vi "RealSense_HelloWorld_PointCloud_ext_RGB2.vi"() -> ()   [LabVIEW 2019]
doc: "Simple Demo showing how to connect a RealSense Camera to stream COLOR and DEPTH from the stereo camera of a D4xx series camera."
uses:
  <vilib>/Utility/miscctls.llb/LV3DPointTypeDef.ctl
  <vilib>/Utility/miscctls.llb/LVRGBAColorTypeDef.ctl
  <vilib>/picture/3D Picture Control/Object/Create Object (name).vi
  Program Files (x86)/RealSense for Labview/RealSense for Labview ver. 2.33/libRealSense3.lvlib
  <vilib>/picture/3D Picture Control/NI_3D Picture Control.lvlib
panel:
  in  "Display tab":T1(tab)=enum."Color + Depth"
  out "RGB height":i32=720
  out "RGB width":i32=1280
  in  "Select RGB Resolution":u16(ring)=28 items=["424 x 240 @6fps", "424 x 240 @15fps", "424 x 240 @30fps", "424 x 240 @60fps", "640 x 480 @6fps", "640 x 480 @15fps", "640 x 480 @30fps", "1280 x 720 @6fps", "1280 x 720 @10fps", "1280 x 720 @15fps", "1920 x 1080 @8fps"]
  out "Depth height":i32=720
  out "Depth width":i32=1280
  out "init results":T2={"camera name"="Intel RealSense D435I", "camera S/N"="834412070342", "F/W"="05.12.01.00", "Sensor name"="Stereo Module", "api_version"=23201, "rscontext"=1659248689968, "device_list"=1659375430384, "device count"=1, "Dev out"=1659375543056, "sensor_list"=1659375327152, "sensor count"=3, "Sensor out"=1659374593968}
  in  "Select Depth Resolution":u16(ring)=29 items=["256 x 144 @90fps", "480 x 270 @6fps", "480 x 270 @15fps", "480 x 270 @30fps", "480 x 270 @60fps", "640 x 360 @30fps", "640 x 480 @6fps", "640 x 480 @15fps", "640 x 480 @30fps", "848 x 480 @6fps", "848 x 480 @8fps", "848 x 480 @10fps", "1280 x 720 @6fps"]
  in  "Sensor index":i32
  in  "Device index":i32
  out "L-R Baseline, mm":sgl=-49.906834
  out "fy":sgl=656.61536 format="%#_5g"
  out "fx":sgl=656.61536 format="%#_5g"
  out "ppy":sgl=357.01468 format="%#_5g"
  out "ppx":sgl=632.28015 format="%#_5g"
  out "RGB Sensor":T3={"Sensor info"="RGB Camera", "Sensor out"=1659374594288, "error"=0}
  out "Stream Profile Handles":u64[](array[numeric])=[1659375449352]
  out "queue out":u64=1659245873280
  out "sensor out":u64=1659374594288
  out "Sensor out":u64=1659374594288
  out "Stream type":u16(ring)=2 items=["Depth"=0, "Color (ext.)"=2, "Color (left) "=3, "IR Left"=5, "IR Right"=9, "IR Left (Y16)"=21, "IR Right (Y16)"=25]
  in  "Exposure,us":sgl=33000.0
  in  "Autoexposure":bool=TRUE
  in  "Depth Presets":T4(ring)=enum."Short Range"
  in  "Color Presets":T5(ring)=enum."D435"
  in  "Laser on/off":bool=TRUE
  in  "Gain(16-248)":sgl=30.0 min=16 max=248
  in  "Update Presets":bool
  in  "Laser \nPower (mW)":dbl(slide)=155.72448 min=0.0 max=360.0 scale=0.36..360.0
  in  "Range Scale":enum16{"200m", "100m", "60m", "6m", "2m", "1m"}(ring)=enum."6m"
  out "RGB image":picture
  out "Depth map":sgl[][](graph)
  out "3D Picture":refnum<vi>(3d-picture)
  out "init error":string="\rNo Error\rNo Error\rNo Error\rNo Error\rNo Error\rNo Error\rNo Error\r\rNo Error\rNo Error"
  out "iteration":i32=762
  in  "stop":bool=TRUE
  # "RealSense Hello World: PointCloud ext. RGB"
  # "This demo shows how to connect a RealSense D435 & D415 Stereo Depth Camera, and display the textured PointCloud."
  # "Note; When you change Depth Preset you need to stop and restart for the HDAD settings to take effect.\n\nTry the Color preset called \"Remove IR2\". It will remove the laser projector from the RGB 1280x720 image."
  # "INTRINSICS & EXTRINSICS"
  # "SELECT THE RESOLUTION"
  # "DEPTH MAP"
  # "COLOR"
  # "Changes Color scale for Depth Map."
  # "20-1660000"
  # "3D POINTCLOUD"
  # "Rotate: Drag image\nMove X-Y: HOLD DOWN CTRL while dragging.\nZoom: SHIFT while dragging."
  # "ERRORS"
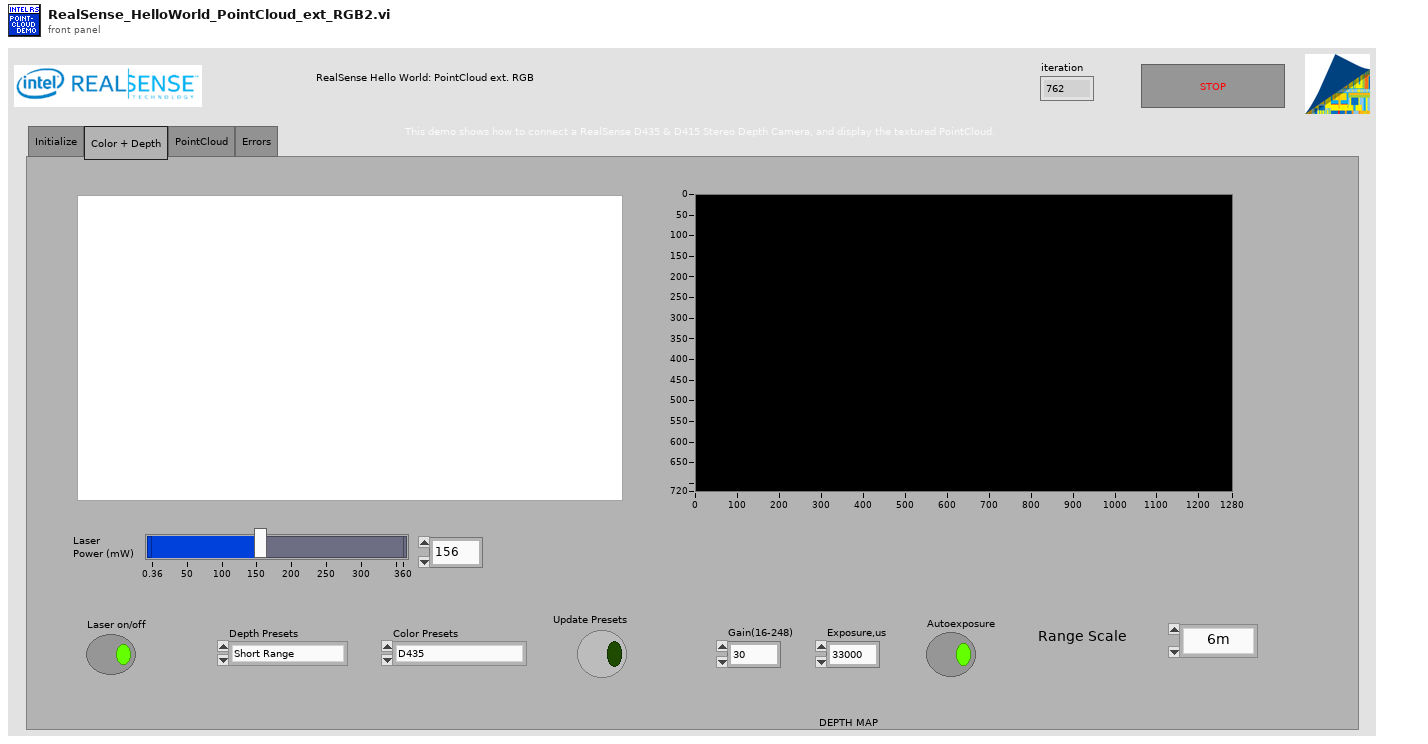
[diagram p1: front panel]
types:
  T1 = enum32{"Initialize", "Color + Depth", "PointCloud", "Errors"}
  T2 = cluster{"camera name":string, "camera S/N":string, "F/W":string, "Sensor name":string, "api_version":i32, "rscontext":u64, "device_list":u64, "device count":i32, "Dev out":u64, "sensor_list":u64, "sensor count":i32, "Sensor out":u64}
  T3 = cluster{"Sensor info":string, "Sensor out":u64, "error":u64}
  T4 = enum16{"Custom", "Original", "New Depth 1", "New Depth 2", "Depth Active 1", "Active 3D Scan", "Active Short A", "Active Short C", "Face", "Face2", "Best Box", "High Density", "Medium Density", "High Accuracy", "Hand", "Short Range", "Flat wall", "Load .JSON", "Load .JSON2"}
  T5 = enum16{"Custom", "RS400 (DS5p)", "RS400 (DS5p) 2", "RS400 (DS5p) 3", "RS400 (DS5p) 4", "RS400 (DS5p) 5", "RS410 (DS5a)", "RS410 (DS5a) 2", "DS410 (DS5a) 3", "DS410 (DS5a) 4", "DS410+IR", "DS5LR", "DS5LR-2", "DS5LR no pattern", "RS410 Remove IR", "RS410 Remove IR 2", "DS5micro", "D435"}
  T6 = cluster{"Sensor info":string, "Sensor out":u64, "error":u64}[]
  T7 = cluster{"width":i32, "height":i32, "fps":i32, "Profile":u64, "ppx":sgl, "ppy":sgl, "fx":sgl, "fy":sgl, "model":u32}
  T8 = enum16{"Overall", "Per Primitive", "Per Vertex", "Binding Off"}
  T9 = enum16{"Points", "Lines", "Line Strip", "Line Loop", "Triangles", "Triangle Strip", "Triangle Fan", "Quads", "Quad Strip", "Polygon"}
  T10 = cluster{"R":dbl, "G":dbl, "B":dbl, "Alpha":dbl}[]
  T11 = typedef "LVRGBAColorTypeDef.ctl" = cluster{"Red":sgl, "Green":sgl, "Blue":sgl, "Alpha":sgl}
  T12 = typedef "LV3DPointTypeDef.ctl" = cluster{"X":sgl, "Y":sgl, "Z":sgl}
  T13 = cluster{"Alpha":sgl, "Blue":sgl, "Green":sgl, "Red":sgl}
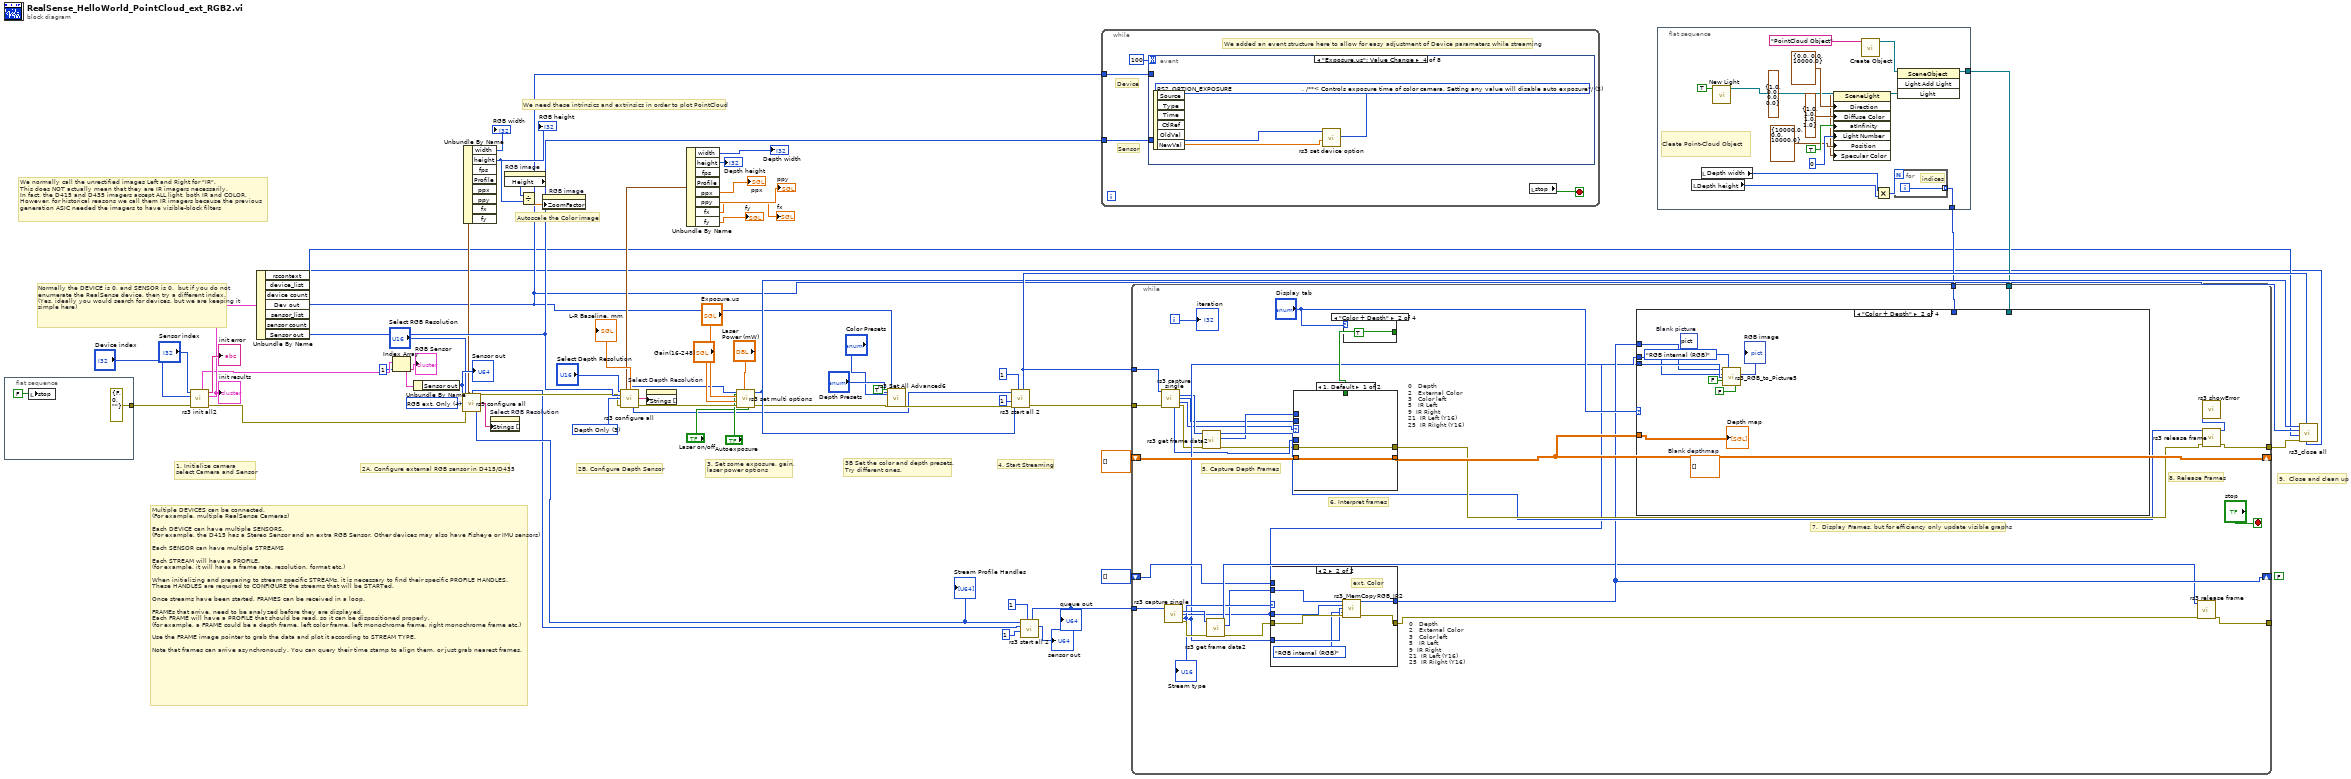
[diagram p0: block diagram]
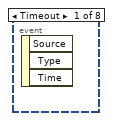
[diagram p2: hidden frame]
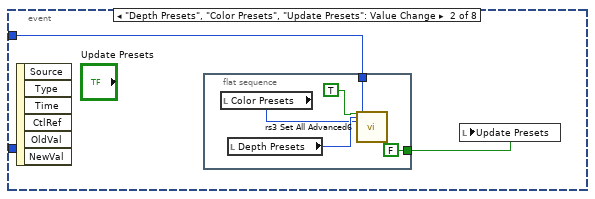
[diagram p3: hidden frame]
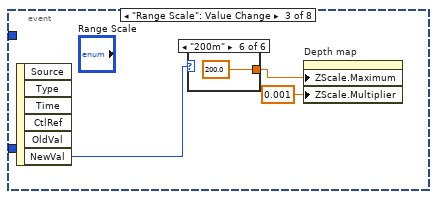
[diagram p4: hidden frame]
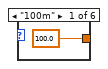
[diagram p5: hidden frame]
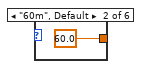
[diagram p6: hidden frame]
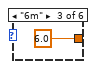
[diagram p7: hidden frame]
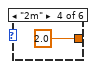
[diagram p8: hidden frame]
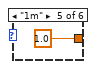
[diagram p9: hidden frame]
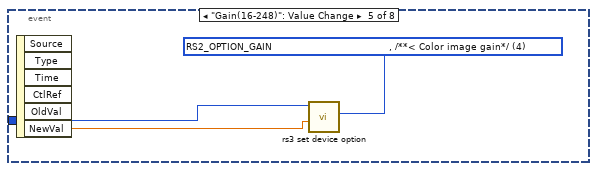
[diagram p10: hidden frame]
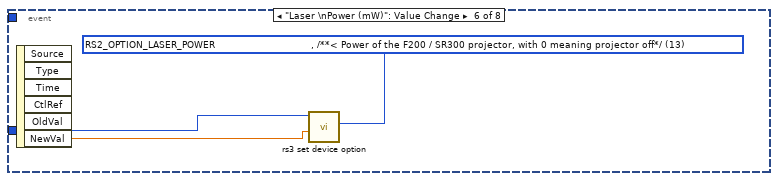
[diagram p11: hidden frame]
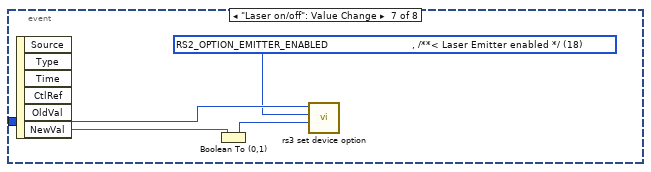
[diagram p12: hidden frame]
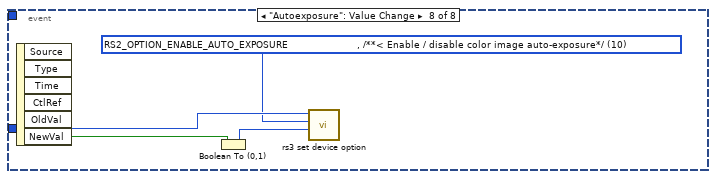
[diagram p13: hidden frame]
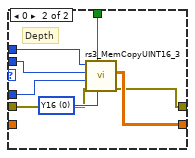
[diagram p14: hidden frame]
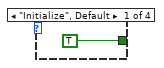
[diagram p16: hidden frame]
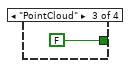
[diagram p17: hidden frame]
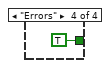
[diagram p18: hidden frame]
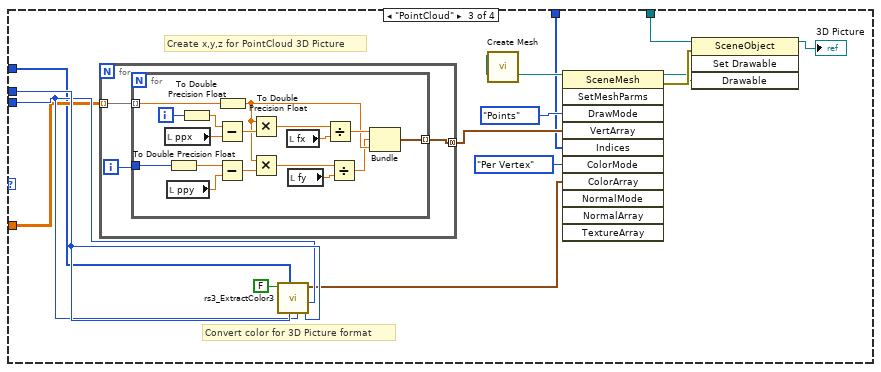
[diagram p20: hidden frame]
diagram:
  (unwired) FALSE
  w16 = u16 4 items=["Depth + Left Color", "Unrectified L + R", "Rectified L + R", "Depth Only", "RGB ext. Only"] ("Stream selection")
  w53 = u16 3 items=["Depth + Left Color", "Unrectified L + R", "Rectified L + R", "Depth Only", "RGB ext. Only"] ("Stream selection")
  # "2A. Configure external RGB sensor in D415/D435"
  # "Autoscale the Color image"
  # "We need these intrinsics and extrinsics in order to plot PointCloud"
  # "3B Set the color and depth presets.\nTry different ones."
  # "We normally call the unrectified images Left and Right for \"IR\". \nThis does NOT actually mean that they are IR imagers necessarily. \nIn fact, the D415 and D435 imagers accept ALL light, both IR and COLOR.\nHowever, for historical reasons we call them IR imagers because the previous generation ASIC needed the imagers to have visible-block filters"
  # "Normally the DEVICE is 0, and SENSOR is 0,  but if you do not enumerate the RealSense device, then try a different index.\n(Yes, ideally you would search for devices, but we are keeping it simple here)"
  # "Multiple DEVICES can be connected. \n(For example, multiple RealSense Cameras)\n\nEach DEVICE can have multiple SENSORS. \n(For example, the D415 has a Stereo Sensor and an extra RGB Sensor. Other devices may also have Fisheye or IMU sensors) \n\nEach SENSOR can have multiple STREAMS\n\nEach STREAM will have a PROFILE. \n(for example, it will have a frame rate, resolution, format etc.)\n\nWhen initializing and preparing to stream specific STREAMs, it is necessary to find their specific PROFILE HANDLES.\nThese HANDLES are required to CONFIGURE the streams that will be STARTed. \n\nOnce streams have been started, FRAMES can be received in a loop. \n \nFRAMEs that arrive, need to be analyzed before they are displayed. \nEach FRAME will have a PROFILE that should be read, so it can be dispositioned properly.\n(for example, a FRAME could be a depth frame, left color frame, left monochrome frame, right monochrome frame etc.)\n\nUse the FRAME image pointer to grab the data and plot it according to STREAM TYPE.\n\nNote that frames can arrive asynchronously. You can query their time stamp to align them, or just grab nearest frames."
  # "9.  Close and clean up"
  # "4. Start Streaming"
  # "3. Set some exposure, gain, \nlaser power options"
  # "2B. Configure Depth Sensor"
  # "1. Initialize camera\nselect Camera and Sensor"
  n1 = flat-sequence {
    tunnel: [errorcluster {"status"=FALSE, "code"=0, "source"=""} ("error in")] -> w54
    frame #0 {
      n2 = local write "stop"(FALSE ("stop")) -> ()
    }
  }
  n3 = call "rs3 init all2.vi"("error in"=w54, "Select Device"="Device index", "Select Sensor"="Sensor index") -> ("error out"=w22:errorcluster, "init results"=w58:T2, "init error"=→"init error":string, "Sensor Array"=w26:T6)  [unwired: 2 in, 3 out]
  "init results" <- w58
  n4 = Unbundle By Name(w58) -> ("rscontext"=w4:u64, "device_list"=w6:u64, "Dev out"=w7:u64, "Sensor out"=w41:u64)  [unwired: 3 out]
  n5 = Index Array(array=w26, index=1) -> (element=w24:T3)
  "RGB Sensor" <- w24
  n6 = Unbundle By Name(w24) -> ("Sensor out"=w23:u64)
  "Sensor out" <- w23
  n7 = call "rs3 configure all.vi"("Select Resolution"="Select RGB Resolution", "Sensor in"=w23, "Stream selection"=w16, "error in (no error)"=w22) -> ("Output stream L"=w19:T7, "Sensor out"=w13:u64, "Output stream"=w3:string[], "Stream Profile Handles"=w14:u64[], "error out"=w20:errorcluster)  [unwired: 2 in, 5 out]
  "Stream Profile Handles" <- w14
  n8 = Unbundle By Name(w19) -> ("width"=→"RGB width":i32, "height"=w17:i32)  [unwired: 6 out]
  "RGB height" <- w17
  n9 = property on="Select RGB Resolution" class="Ring (strict)"("Strings []"=w3) -> ()  [unwired: 2 in, 2 out]
  n10 = property on="RGB image" class="Pict"() -> ("Height"=w37:u32)  [unwired: 2 in, 2 out]
  n11 = Divide(x=w37, y=w17) -> (x/y=w35:dbl)
  n12 = property on="RGB image" class="Pict"("ZoomFactor"=w35) -> ()  [unwired: 2 in, 2 out]
  n13 = call "rs3 configure all.vi"("Select Resolution"="Select Depth Resolution", "Sensor in"=w41, "Stream selection"=w53, "error in (no error)"=w20) -> ("Output stream L"=w38:T7, "Sensor out"=w27:u64, "Output stream"=w55:string[], "L-R Baseline, mm"=→"L-R Baseline, mm":sgl, "Stream Profile Handles"=w15:u64[], "error out"=w52:errorcluster)  [unwired: 2 in, 4 out]
  n14 = property on="Select Depth Resolution" class="Ring (strict)"("Strings []"=w55) -> ()  [unwired: 2 in, 2 out]
  n15 = Unbundle By Name(w38) -> ("width"=→"Depth width":i32, "height"=→"Depth height":i32, "ppx"=→"ppx":sgl, "ppy"=→"ppy":sgl, "fx"=→"fx":sgl, "fy"=→"fy":sgl)  [unwired: 2 out]
  n16 = call "rs3 set multi options.vi"("laser on/off"="Laser on/off", "autoexposure"="Autoexposure", "Laser power, mW (0-360)"="Laser \nPower (mW)", "error in (no error)"=w52, "Gain(16-248)"="Gain(16-248)", "Exposure, us"="Exposure,us", "Sensor in"=w27) -> ("error out"=w46:errorcluster, "Sensor out"=w51:u64)  [unwired: 2 in, 1 out]
  n17 = call "rs3 Set All Advanced6.vi"("Set Color Corr"=TRUE, "Depth Presets"="Depth Presets", "Color Presets"="Color Presets", "error in (no error)"=w46, "device in"=w7) -> ("error out"=w45:errorcluster)  [unwired: 20 in, 2 out]
  n18 = call "rs3 start all 2.vi"("capacity"=1, "error in (no error)"=w45, "Count of Streams"=1, "Sensor in"=w51, "Stream profile array"=w15) -> ("error out"=w56:errorcluster, "queue out"=w61:u64)  [unwired: 3 in, 2 out]
  n19 = call "rs3 start all 2.vi"("capacity"=1, "Count of Streams"=1, "Sensor in"=w13, "Stream profile array"=w14) -> ("sensor out"=→"sensor out":u64, "queue out"=w5:u64)  [unwired: 4 in, 2 out]
  "queue out" <- w5
  n20 = while {
    tunnel: w7 -> [w68]
    tunnel: w41 -> [w67]
    stop <- w69 stop-if-true
    # "Sensor"
    # "Device"
    # "We added an event structure here to allow for easy adjustment of Device parameters while streaming"
    n21 = event shown="[3] \"Exposure,us\": Value Change" {
      selector: _ -> [_ _ _ _ _ _ _ _]
      dyn-events: _ -> [_ _ _ _ _ _ _ _]
      timeout: 100 -> [_ _ _ _ _ _ _ _]
      tunnel: w68 -> [_ w71 _ _ _ _ _ _]
      tunnel: w67 -> [_ _ _ w88 w91 w94 w98 w102]
      event Timeout {
        n22 = event-data() -> ()  [unwired: 1 in, 3 out]
      }
      event "Depth Presets", "Color Presets", "Update Presets": Value Change {
        n23 = event-data() -> ()  [unwired: 1 in, 6 out]
        n24 = flat-sequence {
          tunnel: w71 -> [w73]
          tunnel: [FALSE ("Update Presets")] -> w70
          frame #0 {
            n25 = local read "Color Presets"() -> (w75:T5)
            n26 = local read "Depth Presets"() -> (w76:T4)
            n27 = call "rs3 Set All Advanced6.vi"("Set Color Corr"=TRUE, "Depth Presets"=w76, "Color Presets"=w75, "device in"=w73) -> ()  [unwired: 21 in, 3 out]
          }
        }
        n28 = local write "Update Presets"(w70) -> ()
      }
      event "Range Scale": Value Change {
        n29 = event-data() -> ("NewVal"=w78:enum16{"200m", "100m", "60m", "6m", "2m", "1m"})  [unwired: 1 in, 5 out]
        n30 = case shown="\"200m\"" w78 {
          tunnel: [100.0 ("Z Scale.Offset and Multiplier:Multiplier") 60.0 ("Z Scale.Offset and Multiplier:Multiplier") 6.0 ("Z Scale.Offset and Multiplier:Multiplier") 2.0 ("Z Scale.Offset and Multiplier:Multiplier") 1.0 ("Z Scale.Offset and Multiplier:Multiplier") 200.0 ("Z Scale.Offset and Multiplier:Multiplier")] -> w77
          frame "100m" {
          }
          frame "60m", Default {
          }
          frame "6m" {
          }
          frame "2m" {
          }
          frame "1m" {
          }
          frame "200m" {
          }
        }
        n31 = property on="Depth map" class="IntGraph (strict)"("ZScale.Maximum"=w77, "ZScale.Multiplier"=0.001 ("Z Scale.Offset and Multiplier:Multiplier")) -> ()  [unwired: 2 in, 2 out]
      }
      event "Exposure,us": Value Change {
        w86 = u16 3 items=["    RS2_OPTION_BACKLIGHT_COMPENSATION                     , /**< Enable / disable color backlight compensation*/", "    RS2_OPTION_BRIGHTNESS                                 , /**< Color image brightness*/", "    RS2_OPTION_CONTRAST                                   , /**< Color image contrast*/", "    RS2_OPTION_EXPOSURE                                   , /**< Controls exposure time of color camera. Setting any value will disable auto exposure*/", "    RS2_OPTION_GAIN                                       , /**< Color image gain*/", "    RS2_OPTION_GAMMA                                      , /**< Color image gamma setting*/", "    RS2_OPTION_HUE                                        , /**< Color image hue*/", "    RS2_OPTION_SATURATION                                 , /**< Color image saturation setting*/", "    RS2_OPTION_SHARPNESS                                  , /**< Color image sharpness setting*/", "    RS2_OPTION_WHITE_BALANCE                              , /**< Controls white balance of color image. Setting any value will disable auto white balance*/", "    RS2_OPTION_ENABLE_AUTO_EXPOSURE                       , /**< Enable / disable color image auto-exposure*/", "    RS2_OPTION_ENABLE_AUTO_WHITE_BALANCE                  , /**< Enable / disable color image auto-white-balance*/", "    RS2_OPTION_VISUAL_PRESET                              , /**< Provide access to several recommend sets of option presets for the depth camera */", "    RS2_OPTION_LASER_POWER                                , /**< Power of the F200 / SR300 projector, with 0 meaning projector off*/", "    RS2_OPTION_ACCURACY                                   , /**< Set the number of patterns projected per frame. The higher the accuracy value the more patterns projected. Increasing the number of patterns help to achieve better accuracy. Note that this c", "    RS2_OPTION_MOTION_RANGE                               , /**< Motion vs. Range trade-off, with lower values allowing for better motion sensitivity and higher values allowing for better depth range*/", "    RS2_OPTION_FILTER_OPTION                              , /**< Set the filter to apply to each depth frame. Each one of the filter is optimized per the application requirements*/", "    RS2_OPTION_CONFIDENCE_THRESHOLD                       , /**< The confidence level threshold used by the Depth algorithm pipe to set whether a pixel will get a valid range or will be marked with invalid range*/", "    RS2_OPTION_EMITTER_ENABLED                            , /**< Laser Emitter enabled */", "    RS2_OPTION_FRAMES_QUEUE_SIZE                          , /**< Number of frames the user is allowed to keep per stream. Trying to hold-on to more frames will cause frame-drops.*/", "    RS2_OPTION_TOTAL_FRAME_DROPS                          , /**< Total number of detected frame drops from all streams */", "    RS2_OPTION_AUTO_EXPOSURE_MODE                         , /**< Auto-Exposure modes: Static, Anti-Flicker and Hybrid */", "    RS2_OPTION_POWER_LINE_FREQUENCY                       , /**< Power Line Frequency control for anti-flickering Off/50Hz/60Hz/Auto */", "    RS2_OPTION_ASIC_TEMPERATURE                           , /**< Current Asic Temperature */", "    RS2_OPTION_ERROR_POLLING_ENABLED                      , /**< disable error handling */", "    RS2_OPTION_PROJECTOR_TEMPERATURE                      , /**< Current Projector Temperature */", "    RS2_OPTION_OUTPUT_TRIGGER_ENABLED                     , /**< Enable / disable trigger to be outputed from the camera to any external device on every depth frame */", "    RS2_OPTION_MOTION_MODULE_TEMPERATURE                  , /**< Current Motion-Module Temperature */", "    RS2_OPTION_DEPTH_UNITS                                , /**< Number of meters represented by a single depth unit */", "    RS2_OPTION_ENABLE_MOTION_CORRECTION                   , /**< Enable/Disable automatic correction of the motion data */", "    RS2_OPTION_AUTO_EXPOSURE_PRIORITY                     , /**< Allows sensor to dynamically ajust the frame rate depending on lighting conditions */", "    RS2_OPTION_COUNT                                      , /**< Number of enumeration values. Not a valid input: intended to be used in for-loops. */"] ("RS Option")
        n32 = event-data() -> ("NewVal"=w87:sgl)  [unwired: 1 in, 5 out]
        n33 = call "rs3 set device option.vi"("value"=w87, "RS Option"=w86, "Sensor in"=w88) -> ()  [unwired: 6 in, 3 out]
      }
      event "Gain(16-248)": Value Change {
        w89 = u16 4 items=["    RS2_OPTION_BACKLIGHT_COMPENSATION                     , /**< Enable / disable color backlight compensation*/", "    RS2_OPTION_BRIGHTNESS                                 , /**< Color image brightness*/", "    RS2_OPTION_CONTRAST                                   , /**< Color image contrast*/", "    RS2_OPTION_EXPOSURE                                   , /**< Controls exposure time of color camera. Setting any value will disable auto exposure*/", "    RS2_OPTION_GAIN                                       , /**< Color image gain*/", "    RS2_OPTION_GAMMA                                      , /**< Color image gamma setting*/", "    RS2_OPTION_HUE                                        , /**< Color image hue*/", "    RS2_OPTION_SATURATION                                 , /**< Color image saturation setting*/", "    RS2_OPTION_SHARPNESS                                  , /**< Color image sharpness setting*/", "    RS2_OPTION_WHITE_BALANCE                              , /**< Controls white balance of color image. Setting any value will disable auto white balance*/", "    RS2_OPTION_ENABLE_AUTO_EXPOSURE                       , /**< Enable / disable color image auto-exposure*/", "    RS2_OPTION_ENABLE_AUTO_WHITE_BALANCE                  , /**< Enable / disable color image auto-white-balance*/", "    RS2_OPTION_VISUAL_PRESET                              , /**< Provide access to several recommend sets of option presets for the depth camera */", "    RS2_OPTION_LASER_POWER                                , /**< Power of the F200 / SR300 projector, with 0 meaning projector off*/", "    RS2_OPTION_ACCURACY                                   , /**< Set the number of patterns projected per frame. The higher the accuracy value the more patterns projected. Increasing the number of patterns help to achieve better accuracy. Note that this c", "    RS2_OPTION_MOTION_RANGE                               , /**< Motion vs. Range trade-off, with lower values allowing for better motion sensitivity and higher values allowing for better depth range*/", "    RS2_OPTION_FILTER_OPTION                              , /**< Set the filter to apply to each depth frame. Each one of the filter is optimized per the application requirements*/", "    RS2_OPTION_CONFIDENCE_THRESHOLD                       , /**< The confidence level threshold used by the Depth algorithm pipe to set whether a pixel will get a valid range or will be marked with invalid range*/", "    RS2_OPTION_EMITTER_ENABLED                            , /**< Laser Emitter enabled */", "    RS2_OPTION_FRAMES_QUEUE_SIZE                          , /**< Number of frames the user is allowed to keep per stream. Trying to hold-on to more frames will cause frame-drops.*/", "    RS2_OPTION_TOTAL_FRAME_DROPS                          , /**< Total number of detected frame drops from all streams */", "    RS2_OPTION_AUTO_EXPOSURE_MODE                         , /**< Auto-Exposure modes: Static, Anti-Flicker and Hybrid */", "    RS2_OPTION_POWER_LINE_FREQUENCY                       , /**< Power Line Frequency control for anti-flickering Off/50Hz/60Hz/Auto */", "    RS2_OPTION_ASIC_TEMPERATURE                           , /**< Current Asic Temperature */", "    RS2_OPTION_ERROR_POLLING_ENABLED                      , /**< disable error handling */", "    RS2_OPTION_PROJECTOR_TEMPERATURE                      , /**< Current Projector Temperature */", "    RS2_OPTION_OUTPUT_TRIGGER_ENABLED                     , /**< Enable / disable trigger to be outputed from the camera to any external device on every depth frame */", "    RS2_OPTION_MOTION_MODULE_TEMPERATURE                  , /**< Current Motion-Module Temperature */", "    RS2_OPTION_DEPTH_UNITS                                , /**< Number of meters represented by a single depth unit */", "    RS2_OPTION_ENABLE_MOTION_CORRECTION                   , /**< Enable/Disable automatic correction of the motion data */", "    RS2_OPTION_AUTO_EXPOSURE_PRIORITY                     , /**< Allows sensor to dynamically ajust the frame rate depending on lighting conditions */", "    RS2_OPTION_COUNT                                      , /**< Number of enumeration values. Not a valid input: intended to be used in for-loops. */"] ("RS Option")
        n34 = event-data() -> ("NewVal"=w90:sgl)  [unwired: 1 in, 5 out]
        n35 = call "rs3 set device option.vi"("value"=w90, "RS Option"=w89, "Sensor in"=w91) -> ()  [unwired: 6 in, 3 out]
      }
      event "Laser \nPower (mW)": Value Change {
        w92 = u16 13 items=["    RS2_OPTION_BACKLIGHT_COMPENSATION                     , /**< Enable / disable color backlight compensation*/", "    RS2_OPTION_BRIGHTNESS                                 , /**< Color image brightness*/", "    RS2_OPTION_CONTRAST                                   , /**< Color image contrast*/", "    RS2_OPTION_EXPOSURE                                   , /**< Controls exposure time of color camera. Setting any value will disable auto exposure*/", "    RS2_OPTION_GAIN                                       , /**< Color image gain*/", "    RS2_OPTION_GAMMA                                      , /**< Color image gamma setting*/", "    RS2_OPTION_HUE                                        , /**< Color image hue*/", "    RS2_OPTION_SATURATION                                 , /**< Color image saturation setting*/", "    RS2_OPTION_SHARPNESS                                  , /**< Color image sharpness setting*/", "    RS2_OPTION_WHITE_BALANCE                              , /**< Controls white balance of color image. Setting any value will disable auto white balance*/", "    RS2_OPTION_ENABLE_AUTO_EXPOSURE                       , /**< Enable / disable color image auto-exposure*/", "    RS2_OPTION_ENABLE_AUTO_WHITE_BALANCE                  , /**< Enable / disable color image auto-white-balance*/", "    RS2_OPTION_VISUAL_PRESET                              , /**< Provide access to several recommend sets of option presets for the depth camera */", "    RS2_OPTION_LASER_POWER                                , /**< Power of the F200 / SR300 projector, with 0 meaning projector off*/", "    RS2_OPTION_ACCURACY                                   , /**< Set the number of patterns projected per frame. The higher the accuracy value the more patterns projected. Increasing the number of patterns help to achieve better accuracy. Note that this c", "    RS2_OPTION_MOTION_RANGE                               , /**< Motion vs. Range trade-off, with lower values allowing for better motion sensitivity and higher values allowing for better depth range*/", "    RS2_OPTION_FILTER_OPTION                              , /**< Set the filter to apply to each depth frame. Each one of the filter is optimized per the application requirements*/", "    RS2_OPTION_CONFIDENCE_THRESHOLD                       , /**< The confidence level threshold used by the Depth algorithm pipe to set whether a pixel will get a valid range or will be marked with invalid range*/", "    RS2_OPTION_EMITTER_ENABLED                            , /**< Laser Emitter enabled */", "    RS2_OPTION_FRAMES_QUEUE_SIZE                          , /**< Number of frames the user is allowed to keep per stream. Trying to hold-on to more frames will cause frame-drops.*/", "    RS2_OPTION_TOTAL_FRAME_DROPS                          , /**< Total number of detected frame drops from all streams */", "    RS2_OPTION_AUTO_EXPOSURE_MODE                         , /**< Auto-Exposure modes: Static, Anti-Flicker and Hybrid */", "    RS2_OPTION_POWER_LINE_FREQUENCY                       , /**< Power Line Frequency control for anti-flickering Off/50Hz/60Hz/Auto */", "    RS2_OPTION_ASIC_TEMPERATURE                           , /**< Current Asic Temperature */", "    RS2_OPTION_ERROR_POLLING_ENABLED                      , /**< disable error handling */", "    RS2_OPTION_PROJECTOR_TEMPERATURE                      , /**< Current Projector Temperature */", "    RS2_OPTION_OUTPUT_TRIGGER_ENABLED                     , /**< Enable / disable trigger to be outputed from the camera to any external device on every depth frame */", "    RS2_OPTION_MOTION_MODULE_TEMPERATURE                  , /**< Current Motion-Module Temperature */", "    RS2_OPTION_DEPTH_UNITS                                , /**< Number of meters represented by a single depth unit */", "    RS2_OPTION_ENABLE_MOTION_CORRECTION                   , /**< Enable/Disable automatic correction of the motion data */", "    RS2_OPTION_AUTO_EXPOSURE_PRIORITY                     , /**< Allows sensor to dynamically ajust the frame rate depending on lighting conditions */", "    RS2_OPTION_COUNT                                      , /**< Number of enumeration values. Not a valid input: intended to be used in for-loops. */"] ("RS Option")
        n36 = event-data() -> ("NewVal"=w93:dbl)  [unwired: 1 in, 5 out]
        n37 = call "rs3 set device option.vi"("value"=w93, "RS Option"=w92, "Sensor in"=w94) -> ()  [unwired: 6 in, 3 out]
      }
      event "Laser on/off": Value Change {
        w97 = u16 18 items=["    RS2_OPTION_BACKLIGHT_COMPENSATION                     , /**< Enable / disable color backlight compensation*/", "    RS2_OPTION_BRIGHTNESS                                 , /**< Color image brightness*/", "    RS2_OPTION_CONTRAST                                   , /**< Color image contrast*/", "    RS2_OPTION_EXPOSURE                                   , /**< Controls exposure time of color camera. Setting any value will disable auto exposure*/", "    RS2_OPTION_GAIN                                       , /**< Color image gain*/", "    RS2_OPTION_GAMMA                                      , /**< Color image gamma setting*/", "    RS2_OPTION_HUE                                        , /**< Color image hue*/", "    RS2_OPTION_SATURATION                                 , /**< Color image saturation setting*/", "    RS2_OPTION_SHARPNESS                                  , /**< Color image sharpness setting*/", "    RS2_OPTION_WHITE_BALANCE                              , /**< Controls white balance of color image. Setting any value will disable auto white balance*/", "    RS2_OPTION_ENABLE_AUTO_EXPOSURE                       , /**< Enable / disable color image auto-exposure*/", "    RS2_OPTION_ENABLE_AUTO_WHITE_BALANCE                  , /**< Enable / disable color image auto-white-balance*/", "    RS2_OPTION_VISUAL_PRESET                              , /**< Provide access to several recommend sets of option presets for the depth camera */", "    RS2_OPTION_LASER_POWER                                , /**< Power of the F200 / SR300 projector, with 0 meaning projector off*/", "    RS2_OPTION_ACCURACY                                   , /**< Set the number of patterns projected per frame. The higher the accuracy value the more patterns projected. Increasing the number of patterns help to achieve better accuracy. Note that this c", "    RS2_OPTION_MOTION_RANGE                               , /**< Motion vs. Range trade-off, with lower values allowing for better motion sensitivity and higher values allowing for better depth range*/", "    RS2_OPTION_FILTER_OPTION                              , /**< Set the filter to apply to each depth frame. Each one of the filter is optimized per the application requirements*/", "    RS2_OPTION_CONFIDENCE_THRESHOLD                       , /**< The confidence level threshold used by the Depth algorithm pipe to set whether a pixel will get a valid range or will be marked with invalid range*/", "    RS2_OPTION_EMITTER_ENABLED                            , /**< Laser Emitter enabled */", "    RS2_OPTION_FRAMES_QUEUE_SIZE                          , /**< Number of frames the user is allowed to keep per stream. Trying to hold-on to more frames will cause frame-drops.*/", "    RS2_OPTION_TOTAL_FRAME_DROPS                          , /**< Total number of detected frame drops from all streams */", "    RS2_OPTION_AUTO_EXPOSURE_MODE                         , /**< Auto-Exposure modes: Static, Anti-Flicker and Hybrid */", "    RS2_OPTION_POWER_LINE_FREQUENCY                       , /**< Power Line Frequency control for anti-flickering Off/50Hz/60Hz/Auto */", "    RS2_OPTION_ASIC_TEMPERATURE                           , /**< Current Asic Temperature */", "    RS2_OPTION_ERROR_POLLING_ENABLED                      , /**< disable error handling */", "    RS2_OPTION_PROJECTOR_TEMPERATURE                      , /**< Current Projector Temperature */", "    RS2_OPTION_OUTPUT_TRIGGER_ENABLED                     , /**< Enable / disable trigger to be outputed from the camera to any external device on every depth frame */", "    RS2_OPTION_MOTION_MODULE_TEMPERATURE                  , /**< Current Motion-Module Temperature */", "    RS2_OPTION_DEPTH_UNITS                                , /**< Number of meters represented by a single depth unit */", "    RS2_OPTION_ENABLE_MOTION_CORRECTION                   , /**< Enable/Disable automatic correction of the motion data */", "    RS2_OPTION_AUTO_EXPOSURE_PRIORITY                     , /**< Allows sensor to dynamically ajust the frame rate depending on lighting conditions */", "    RS2_OPTION_COUNT                                      , /**< Number of enumeration values. Not a valid input: intended to be used in for-loops. */"] ("RS Option")
        n38 = event-data() -> ("NewVal"=w96:bool)  [unwired: 1 in, 5 out]
        n39 = Boolean To (0,1)(Boolean=w96) -> (0, 1=w95:i16)
        n40 = call "rs3 set device option.vi"("value"=w95, "RS Option"=w97, "Sensor in"=w98) -> ()  [unwired: 6 in, 3 out]
      }
      event "Autoexposure": Value Change {
        w101 = u16 10 items=["    RS2_OPTION_BACKLIGHT_COMPENSATION                     , /**< Enable / disable color backlight compensation*/", "    RS2_OPTION_BRIGHTNESS                                 , /**< Color image brightness*/", "    RS2_OPTION_CONTRAST                                   , /**< Color image contrast*/", "    RS2_OPTION_EXPOSURE                                   , /**< Controls exposure time of color camera. Setting any value will disable auto exposure*/", "    RS2_OPTION_GAIN                                       , /**< Color image gain*/", "    RS2_OPTION_GAMMA                                      , /**< Color image gamma setting*/", "    RS2_OPTION_HUE                                        , /**< Color image hue*/", "    RS2_OPTION_SATURATION                                 , /**< Color image saturation setting*/", "    RS2_OPTION_SHARPNESS                                  , /**< Color image sharpness setting*/", "    RS2_OPTION_WHITE_BALANCE                              , /**< Controls white balance of color image. Setting any value will disable auto white balance*/", "    RS2_OPTION_ENABLE_AUTO_EXPOSURE                       , /**< Enable / disable color image auto-exposure*/", "    RS2_OPTION_ENABLE_AUTO_WHITE_BALANCE                  , /**< Enable / disable color image auto-white-balance*/", "    RS2_OPTION_VISUAL_PRESET                              , /**< Provide access to several recommend sets of option presets for the depth camera */", "    RS2_OPTION_LASER_POWER                                , /**< Power of the F200 / SR300 projector, with 0 meaning projector off*/", "    RS2_OPTION_ACCURACY                                   , /**< Set the number of patterns projected per frame. The higher the accuracy value the more patterns projected. Increasing the number of patterns help to achieve better accuracy. Note that this c", "    RS2_OPTION_MOTION_RANGE                               , /**< Motion vs. Range trade-off, with lower values allowing for better motion sensitivity and higher values allowing for better depth range*/", "    RS2_OPTION_FILTER_OPTION                              , /**< Set the filter to apply to each depth frame. Each one of the filter is optimized per the application requirements*/", "    RS2_OPTION_CONFIDENCE_THRESHOLD                       , /**< The confidence level threshold used by the Depth algorithm pipe to set whether a pixel will get a valid range or will be marked with invalid range*/", "    RS2_OPTION_EMITTER_ENABLED                            , /**< Laser Emitter enabled */", "    RS2_OPTION_FRAMES_QUEUE_SIZE                          , /**< Number of frames the user is allowed to keep per stream. Trying to hold-on to more frames will cause frame-drops.*/", "    RS2_OPTION_TOTAL_FRAME_DROPS                          , /**< Total number of detected frame drops from all streams */", "    RS2_OPTION_AUTO_EXPOSURE_MODE                         , /**< Auto-Exposure modes: Static, Anti-Flicker and Hybrid */", "    RS2_OPTION_POWER_LINE_FREQUENCY                       , /**< Power Line Frequency control for anti-flickering Off/50Hz/60Hz/Auto */", "    RS2_OPTION_ASIC_TEMPERATURE                           , /**< Current Asic Temperature */", "    RS2_OPTION_ERROR_POLLING_ENABLED                      , /**< disable error handling */", "    RS2_OPTION_PROJECTOR_TEMPERATURE                      , /**< Current Projector Temperature */", "    RS2_OPTION_OUTPUT_TRIGGER_ENABLED                     , /**< Enable / disable trigger to be outputed from the camera to any external device on every depth frame */", "    RS2_OPTION_MOTION_MODULE_TEMPERATURE                  , /**< Current Motion-Module Temperature */", "    RS2_OPTION_DEPTH_UNITS                                , /**< Number of meters represented by a single depth unit */", "    RS2_OPTION_ENABLE_MOTION_CORRECTION                   , /**< Enable/Disable automatic correction of the motion data */", "    RS2_OPTION_AUTO_EXPOSURE_PRIORITY                     , /**< Allows sensor to dynamically ajust the frame rate depending on lighting conditions */", "    RS2_OPTION_COUNT                                      , /**< Number of enumeration values. Not a valid input: intended to be used in for-loops. */"] ("RS Option")
        n41 = event-data() -> ("NewVal"=w100:bool)  [unwired: 1 in, 5 out]
        n42 = Boolean To (0,1)(Boolean=w100) -> (0, 1=w99:i16)
        n43 = call "rs3 set device option.vi"("value"=w99, "RS Option"=w101, "Sensor in"=w102) -> ()  [unwired: 6 in, 3 out]
      }
    }
    n44 = local read "stop"() -> (w69:bool)
  }
  n45 = while {
    tunnel: w61 -> [w133]
    tunnel: w56 -> [w136]
    tunnel: [w134] -> w60
    shift-right: [w126] -> _
    shift-left: sgl[][] [] ("2D Array Output") -> [w131]
    tunnel: w30 -> [w130]
    tunnel: w28 -> [w129]
    tunnel: w5 -> [w123]
    tunnel: [w118] -> _
    shift-right: [w117] -> _
    shift-left: u8[] [] ("Output Array") -> [w115]
    i -> [w135]
    stop <- "stop" stop-if-true
    # "0   Depth\n2   External Color \n3   Color left\n5   IR Left \n9  IR Right\n21  IR Left (Y16)\n25  IR RiIght (Y16)"
    # "0   Depth\n2   External Color \n3   Color left\n5   IR Left \n9  IR Right\n21  IR Left (Y16)\n25  IR RiIght (Y16)"
    # "6. Interpret frames"
    # "5. Capture Depth Frames"
    # "8. Release Frames"
    # "7.  Display Frames, but for efficiency only update visible graphs"
    n46 = call "rs3 capture single.vi"("queue in"=w133, "error in (no error)"=w136) -> ("frame out"=w110:u64, "width"=w107:i32, "Stream type"=w108:u16, "height"=w106:i32, "error out"=w104:errorcluster)  [unwired: 5 in, 4 out]
    n47 = call "rs3 capture single.vi"("queue in"=w123) -> ("frame out"=w121:u64, "width"=w112:i32, "Stream type"=w114:u16, "height"=w111:i32, "error out"=w122:errorcluster)  [unwired: 6 in, 4 out]
    "Stream type" <- w114
    n48 = call "rs3 get frame data2.vi"("error in (no error)"=w104, "frame in"=w110) -> ("error out"=w105:errorcluster, "image pointer out"=w109:u64, "Frame out"=w124:u64)  [unwired: 6 in, 1 out]
    n49 = call "rs3 get frame data2.vi"("error in (no error)"=w122, "frame in"=w121) -> ("error out"=w120:errorcluster, "image pointer out"=w113:u64, "Frame out"=w116:u64)  [unwired: 6 in, 1 out]
    n50 = case shown="2" w114 {
      tunnel: [w148 w154] -> w119
      tunnel: w113 -> [_ w155]
      tunnel: w120 -> [w148 w153]
      tunnel: w112 -> [_ w152]
      tunnel: w111 -> [_ w151]
      tunnel: [w147 w150] -> w117
      tunnel: w115 -> [w147 _]
      frame 1, Default {
      }
      frame 2 {
        # "ext. Color"
        n51 = call "rs3_MemCopyRGB_IR2.vi"("Zimage pointer"=w155, "RGB  X, width"=w152, "RGB Y, height"=w151, "Color format"=enum16{"Monochrome", "RGB internal (RGB)"}."RGB internal (RGB)", "error in (no error)"=w153) -> ("Output Array"=w150:u8[], "error out"=w154:errorcluster)  [unwired: 8 in, 1 out]
      }
    }
    n52 = case shown="\"Color + Depth\"" "Display tab" {
      tunnel: [TRUE ("Transpose") TRUE ("Transpose") FALSE ("Transpose") TRUE ("Transpose")] -> w127
      frame "Initialize", Default {
      }
      frame "Color + Depth" {
      }
      frame "PointCloud" {
      }
      frame "Errors" {
      }
    }
    n53 = case shown="1, Default" w108 {
      tunnel: [w138 w143] -> w125
      tunnel: w109 -> [_ w142]
      tunnel: w107 -> [_ w141]
      tunnel: w106 -> [_ w140]
      tunnel: w105 -> [w138 w144]
      tunnel: [w137 w145] -> w126
      tunnel: w131 -> [w137 _]
      tunnel: w127 -> [_ w139]
      frame 1, Default {
      }
      frame 0 {
        w146 = u16 0 items=["Y16", "Y8"] ("Image format")
        # "Depth"
        n54 = call "rs3_MemCopyUINT16_3.vi"("Image format"=w146, "Transpose"=w139, "error in (no error)"=w144, "Depth Y"=w140, "Depth X"=w141, "Zimage pointer"=w142) -> ("error out"=w143:errorcluster, "2D Array Output"=w145:sgl[][])  [unwired: 2 in, 2 out]
      }
    }
    n55 = case shown="\"Color + Depth\"" "Display tab" {
      tunnel: w112 -> [_ w161 w182 _]
      tunnel: w111 -> [_ w167 w181 _]
      tunnel: w126 -> [_ w166 w169 _]
      tunnel: w130 -> [_ _ w171 _]
      tunnel: w129 -> [_ _ w170 _]
      tunnel: w117 -> [_ w165 w168 _]
      frame "Initialize", Default {
      }
      frame "Color + Depth" {
        (unwired) picture bytes[33]  # Blank picture
        (unwired) sgl[][] []  # Blank depthmap
        n56 = call "rs3_RGB_to_Picture5.vi"("RGB array"=w165, "Color format"=enum16{"Monochrome", "RGB internal (RGB)"}."RGB internal (RGB)", "RGB  X, width"=w161, "RGB Y, height"=w167, "AWB"=FALSE, "White Balance"=FALSE) -> ("new picture"=→"RGB image":picture)  [unwired: 8 in, 1 out]
        "Depth map" <- w166
      }
      frame "PointCloud" {
        # "Convert color for 3D Picture format"
        # "Create x,y,z for PointCloud 3D Picture"
        n57 = for {
          tunnel: w169 -> [w185] mode=indexing
          tunnel: [w184] -> w175 mode=concatenating
          i -> [w183]
          n58 = for {
            tunnel: w185 -> [w202] mode=indexing
            tunnel: w183 -> [w201]
            tunnel: [w200] -> w184 mode=indexing
            i -> [w199]
            n59 = local read "ppx"() -> (w192:sgl)
            n60 = local read "ppy"() -> (w190:sgl)
            n61 = To Double Precision Float(number=w201) -> (double precision float=w189:dbl)
            n62 = To Double Precision Float(number=w199) -> (double precision float=w194:dbl)
            n63 = Subtract(x=w194, y=w192) -> (x-y=w193:dbl)
            n64 = Subtract(x=w189, y=w190) -> (x-y=w188:dbl)
            n65 = To Double Precision Float(number=w202) -> (double precision float=w187:dbl)
            n66 = Multiply(x=w187, y=w193) -> (x*y=w198:dbl)
            n67 = Multiply(x=w187, y=w188) -> (x*y=w195:dbl)
            n68 = local read "fx"() -> (w197:sgl)
            n69 = local read "fy"() -> (w191:sgl)
            n70 = Divide(x=w198, y=w197) -> (x/y=w196:dbl)
            n71 = Divide(x=w195, y=w191) -> (x/y=w186:dbl)
            n72 = Bundle(w196, w186, w187) -> (w200:cluster{dbl, dbl, dbl})  [unwired: 1 in]
          }
        }
        n73 = call "rs3_ExtractColor3.vi"("Depth X"=w182, "Depth Y"=w181, "RGB Y"=w181, "RGB  X"=w182, "24bit Color Array"=w168, "White Balance"=FALSE) -> ("Norm Mesh Color"=w174:T10)  [unwired: 5 in]
        n74 = call <vilib>:"Create Mesh.vi"() -> ("New Mesh Refnum"=w177:refnum<vi>)  [unwired: 10 in, 1 out]
        n75 = invoke class="SceneMesh" method="SetMeshParms"(reference=w177, "DrawMode"=T9."Points" ("Draw Mode"), "VertArray"=w175, "Indices"=w170, "ColorMode"=T8."Per Vertex" ("Color Binding Mode"), "ColorArray"=w174) -> (reference out=w178:refnum<vi>, error out=w179:errorcluster)  [unwired: 5 in, 9 out]
        n76 = invoke class="SceneObject" method="Set Drawable"(reference=w171, error in=w179, "Drawable"=w178) -> (reference out=→"3D Picture":refnum<vi>)  [unwired: 1 in, 3 out]
      }
      frame "Errors" {
      }
    }
    n77 = call "rs3 release frame.vi"("error in (no error)"=w119, "Frame"=w116) -> ("error out"=w118:errorcluster)  [unwired: 8 in, 1 out]
    n78 = call "rs3 release frame.vi"("error in (no error)"=w125, "Frame"=w124) -> ("error out"=w134:errorcluster, "error"=w103:u64)  [unwired: 8 in]
    n79 = call "rs3 showError.vi"("error"=w103) -> ()  [unwired: 6 in, 5 out]
    "iteration" <- w135
  }
  n80 = flat-sequence {
    tunnel: [w207] -> w30
    tunnel: [w203] -> w28
    frame #0 {
      # "Cleate Point-Cloud Object"
      n81 = local read "Depth height"() -> (w204:i32)
      n82 = local read "Depth width"() -> (w205:i32)
      n83 = call <vilib>:"New Light.vi"("At Infinity"=TRUE) -> ("New Light Refnum"=w215:refnum<vi>)  [unwired: 2 in, 8 out]
      n84 = property class="SceneLight"(reference=w215, "Direction"=cluster{"X":sgl, "Y":sgl, "Z":sgl} {"X"=0.0, "Y"=0.0, "Z"=10000.0}, "Diffuse Color"=T13 {"Alpha"=1.0, "Blue"=1.0, "Green"=1.0, "Red"=1.0}, "atInfinity"=TRUE ("At Infinity"), "Light Number"=0, "Position"=T12 {"X"=10000.0, "Y"=0.0, "Z"=10000.0}, "Specular Color"=T11 {"Red"=1.0, "Green"=0.0, "Blue"=0.0, "Alpha"=0.0}) -> (reference out=w212:refnum<vi>)  [unwired: 1 in, 1 out]
      n85 = call-poly <vilib>:"Create Object.vi"("Name"="PointCloud Object") -> ("Scene:New Object"=w214:refnum<vi>)  [unwired: 9 in, 1 out]
      n86 = Multiply(x=w205, y=w204) -> (x*y=w206:i32)
      n87 = for {
        N: w206 -> [_]
        tunnel: [w219] -> w203 mode=indexing
        i -> [w219]
        # "indices"
      }
      n88 = invoke class="SceneObject" method="Light.Add Light"(reference=w214, "Light"=w212) -> (reference out=w207:refnum<vi>)  [unwired: 2 in, 3 out]
    }
  }
  n89 = call "rs3_close all.vi"("rscontext"=w4, "queue in"=w61, "error in (no error)"=w60, "device_list"=w6, "Dev in"=w7, "Sensor in"=w51) -> ()  [unwired: 4 in, 2 out]
